vi "Generate Error.vi"(7 "Mode":T5(ring), 8 "error in (no error)":errorcluster, 11 "Method Result In":T1) -> (0 "error out":errorcluster, 3 "Method Result Out":T1)   [LabVIEW 2020, in "Method Result.lvlib"]
uses:
  Method Result.lvlib
  Assertion Result/Public/TypeDefs/Status.ctl
  Assertion Result/Assertion Result.lvlib
  Assertion Result/Public/TypeDefs/Assertion Type.ctl
  Assertion Result/Assertion Result.ctl
  Method Result.ctl
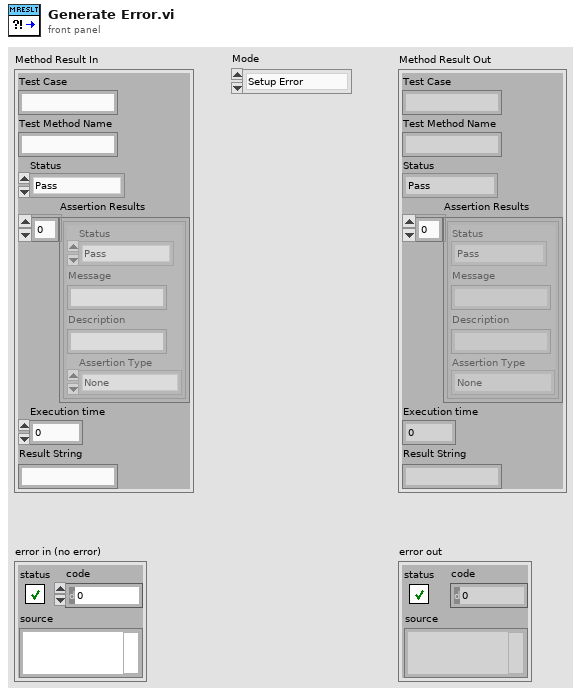
[diagram p1: front panel]
types:
  T1 = typedef "Method Result.lvlib/Method Result.ctl" = cluster{"Test Case":string, "Test Method Name":string, "Status":T2, "Assertion Results":T3[], "Execution time":dbl, "Result String":string}
  T2 = typedef "Assertion Result.lvlib/Status.ctl" = enum16{"Pass", "Fail", "Error", "Skipped", "Setup Error", "Broken", "Teardown Error"}
  T3 = typedef "Assertion Result.lvlib/Assertion Result.ctl" = cluster{"Status":T2, "Message":string, "Description":string, "Assertion Type":T4}
  T4 = typedef "Assertion Result.lvlib/Assertion Type.ctl" = enum16{"None", "Pass", "Fail", "Skip", "Pass if Equal", "Fail if Equal", "Pass if Error", "Fail if Error", "Pass if", "Fail if"}
  T5 = enum16{"Setup Error", "Teardown Error", "Broken", "Test Method Error"}
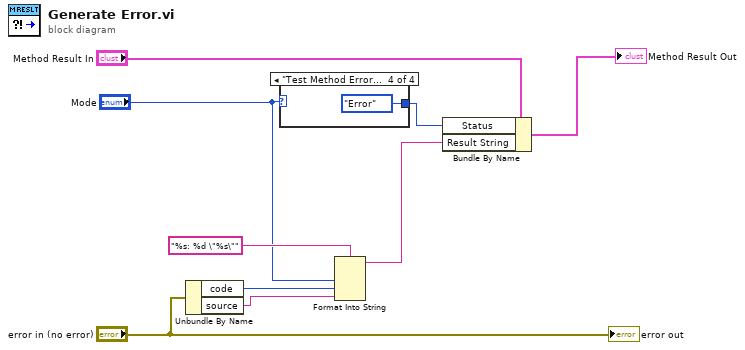
[diagram p0: block diagram]
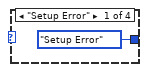
[diagram p2: hidden frame]
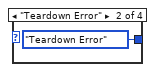
[diagram p3: hidden frame]
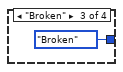
[diagram p4: hidden frame]
diagram:
  n1 = Unbundle By Name("error in (no error)") -> ("code"=w5:i32, "source"=w4:string)
  n2 = case shown="\"Test Method Error\"" "Mode" {
    tunnel: [Status."Setup Error" ("Status") Status."Teardown Error" ("Status") Status."Broken" ("Status") Status."Error" ("Status")] -> w8
    frame "Setup Error" {
    }
    frame "Teardown Error" {
    }
    frame "Broken" {
    }
    frame "Test Method Error" {
    }
  }
  n3 = Format Into String(format string="%s: %d \"%s\"", "Mode", w5, w4) -> (resulting string=w1:string)  [unwired: 2 in, 1 out]
  n4 = Bundle By Name(cluster="Method Result In", "Status"=w8, "Result String"=w1) -> (→"Method Result Out":T1)
  "error out" <- "error in (no error)"
